vi "MultiTool-Track-Generate-ndipolarisFileOutput-Q-vectors-Accepts Joystick mod10Feb2018.vi"() -> ()   [LabVIEW 2013]
panel:
  out "TIME":string
  out "bytes written":i32
  out "Return time string":string
  out "Length":u8
  out "Command":u8
  out "Tool 2":T1={"Port Handle"="", "Frame Number"=0, "Tx"=0.0, "Ty"=0.0, "Tz"=0.0, "Q0"=0.0, "Qx"=0.0, "Qy"=0.0, "Qz"=0.0, "Deviation"=0.0, " Markers Missing"=TRUE, "Out of Volume"=TRUE} {"Deviation" format="%#.4f"; "Qz" format="%#.4f"; "Qy" format="%#.4f"; "Qx" format="%#.4f"; "Q0" format="%#.4f"; "Tz" format="%#.2f"; "Ty" format="%#.2f"; "Tx" format="%#.2f"}
  in  "Location of ROM File for Tool 2":path=path "C:/Program Files (x86)/Northern Digital Inc/8700339.rom"
  in  "NDI  Running":bool=TRUE
  out "Stop Reading":bool=TRUE
  out "Start Reading":bool
  out "Object Identifier":string="0"
  in  "Track Outside Measurement Volume? (F:No)":bool
  in  "Track Stray Markers? (F:No)":bool
  out "Tool 1":T1={"Port Handle"="", "Frame Number"=0, "Tx"=0.0, "Ty"=0.0, "Tz"=0.0, "Q0"=0.0, "Qx"=0.0, "Qy"=0.0, "Qz"=0.0, "Deviation"=0.0, " Markers Missing"=TRUE, "Out of Volume"=TRUE} {"Deviation" format="%#.4f"; "Qz" format="%#.4f"; "Qy" format="%#.4f"; "Qx" format="%#.4f"; "Q0" format="%#.4f"; "Tz" format="%#.2f"; "Ty" format="%#.2f"; "Tx" format="%#.2f"}
  out "TCP loop":i32
  in  "TCP Server Running":bool=TRUE
  in  "Output Directory":path=path "C:/Users/Diogo/Desktop/NDI-Labview Gripper"
  out "NDI Loop":i32
  in  "VISA resource name":refnum<visa-resource-name>="COM8"
  in  "Reset? (T:Yes)":bool=TRUE
  in  "Location of ROM File for Tool 1":path=path "C:/Program Files (x86)/Northern Digital Inc/8700449.rom"
  in  "Serial Configuration":T2={"Baud Rate (9600)"=9600, "Flow Control (0:None)"=0, "Parity"=0, "Data Bits"=8, "Stop Bits"=10} {"Stop Bits" items=["1.0"=10, "2.0"=20]; "Parity" items=["None", "Odd", "Even"]; "Flow Control (0:None)" items=["None", "XON/XOFF"]; "Baud Rate (9600)" items=["9600"=9600, "14.4k"=14400, "19.2k"=19200, "38.4k"=38400, "57.6k "=57600, "115.2k"=115200]}
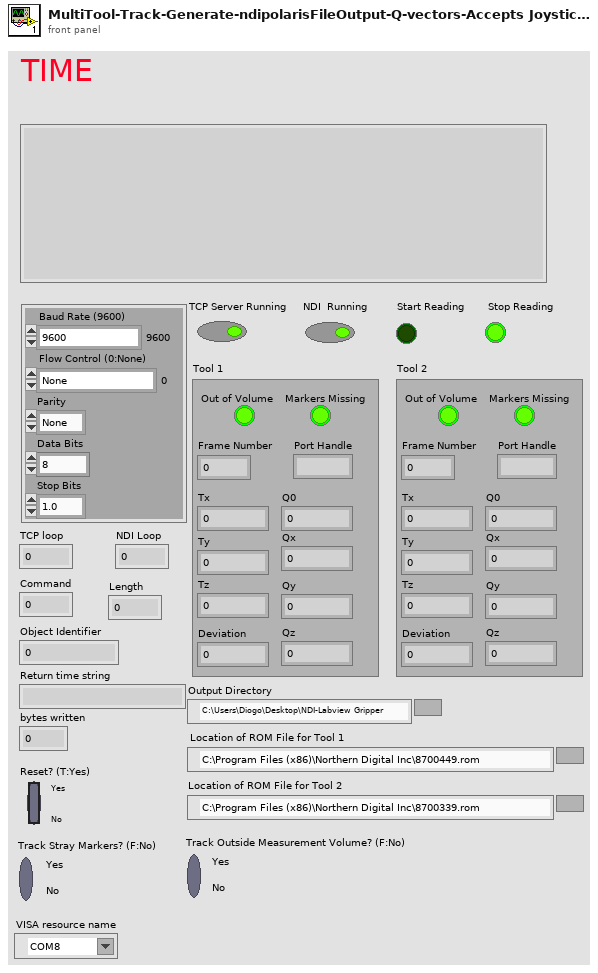
[diagram p1: front panel]
types:
  T1 = cluster{"Port Handle":string, "Frame Number":i32, "Tx":dbl, "Ty":dbl, "Tz":dbl, "Q0":dbl, "Qx":dbl, "Qy":dbl, "Qz":dbl, "Deviation":dbl, " Markers Missing":bool, "Out of Volume":bool}
  T2 = cluster{"Baud Rate (9600)":u32, "Flow Control (0:None)":u16, "Parity":u16, "Data Bits":u16, "Stop Bits":u16}
  T3 = cluster{"Port Handle":string, "Frame Number":u32, "Tx":dbl, "Ty":dbl, "Tz":dbl, "Q0":dbl, "Qx":dbl, "Qy":dbl, "Qz":dbl, "Deviation":dbl, "Missing?":bool, "Out of Volume?":bool}[]
  T4 = cluster{"Transformations[0]":cluster{"Port Handle":string, "Frame Number":u32, "Tx":dbl, "Ty":dbl, "Tz":dbl, "Q0":dbl, "Qx":dbl, "Qy":dbl, "Qz":dbl, "Deviation":dbl, "Missing?":bool, "Out of Volume?":bool}, "Transformations[1]":cluster{"Port Handle":string, "Frame Number":u32, "Tx":dbl, "Ty":dbl, "Tz":dbl, "Q0":dbl, "Qx":dbl, "Qy":dbl, "Qz":dbl, "Deviation":dbl, "Missing?":bool, "Out of Volume?":bool}, "Transformations[2]":cluster{"Port Handle":string, "Frame Number":u32, "Tx":dbl, "Ty":dbl, "Tz":dbl, "Q0":dbl, "Qx":dbl, "Qy":dbl, "Qz":dbl, "Deviation":dbl, "Missing?":bool, "Out of Volume?":bool}, "Transformations[3]":cluster{"Port Handle":string, "Frame Number":u32, "Tx":dbl, "Ty":dbl, "Tz":dbl, "Q0":dbl, "Qx":dbl, "Qy":dbl, "Qz":dbl, "Deviation":dbl, "Missing?":bool, "Out of Volume?":bool}, "Transformations[4]":cluster{"Port Handle":string, "Frame Number":u32, "Tx":dbl, "Ty":dbl, "Tz":dbl, "Q0":dbl, "Qx":dbl, "Qy":dbl, "Qz":dbl, "Deviation":dbl, "Missing?":bool, "Out of Volume?":bool}, "Transformations[5]":cluster{"Port Handle":string, "Frame Number":u32, "Tx":dbl, "Ty":dbl, "Tz":dbl, "Q0":dbl, "Qx":dbl, "Qy":dbl, "Qz":dbl, "Deviation":dbl, "Missing?":bool, "Out of Volume?":bool}, "Transformations[6]":cluster{"Port Handle":string, "Frame Number":u32, "Tx":dbl, "Ty":dbl, "Tz":dbl, "Q0":dbl, "Qx":dbl, "Qy":dbl, "Qz":dbl, "Deviation":dbl, "Missing?":bool, "Out of Volume?":bool}, "Transformations[7]":cluster{"Port Handle":string, "Frame Number":u32, "Tx":dbl, "Ty":dbl, "Tz":dbl, "Q0":dbl, "Qx":dbl, "Qy":dbl, "Qz":dbl, "Deviation":dbl, "Missing?":bool, "Out of Volume?":bool}, "Transformations[8]":cluster{"Port Handle":string, "Frame Number":u32, "Tx":dbl, "Ty":dbl, "Tz":dbl, "Q0":dbl, "Qx":dbl, "Qy":dbl, "Qz":dbl, "Deviation":dbl, "Missing?":bool, "Out of Volume?":bool}}
  T5 = cluster{"Port Handle":string, "Frame Number":u32, "Tx":dbl, "Ty":dbl, "Tz":dbl, "Q0":dbl, "Qx":dbl, "Qy":dbl, "Qz":dbl, "Deviation":dbl, "Missing?":bool, "Out of Volume?":bool}
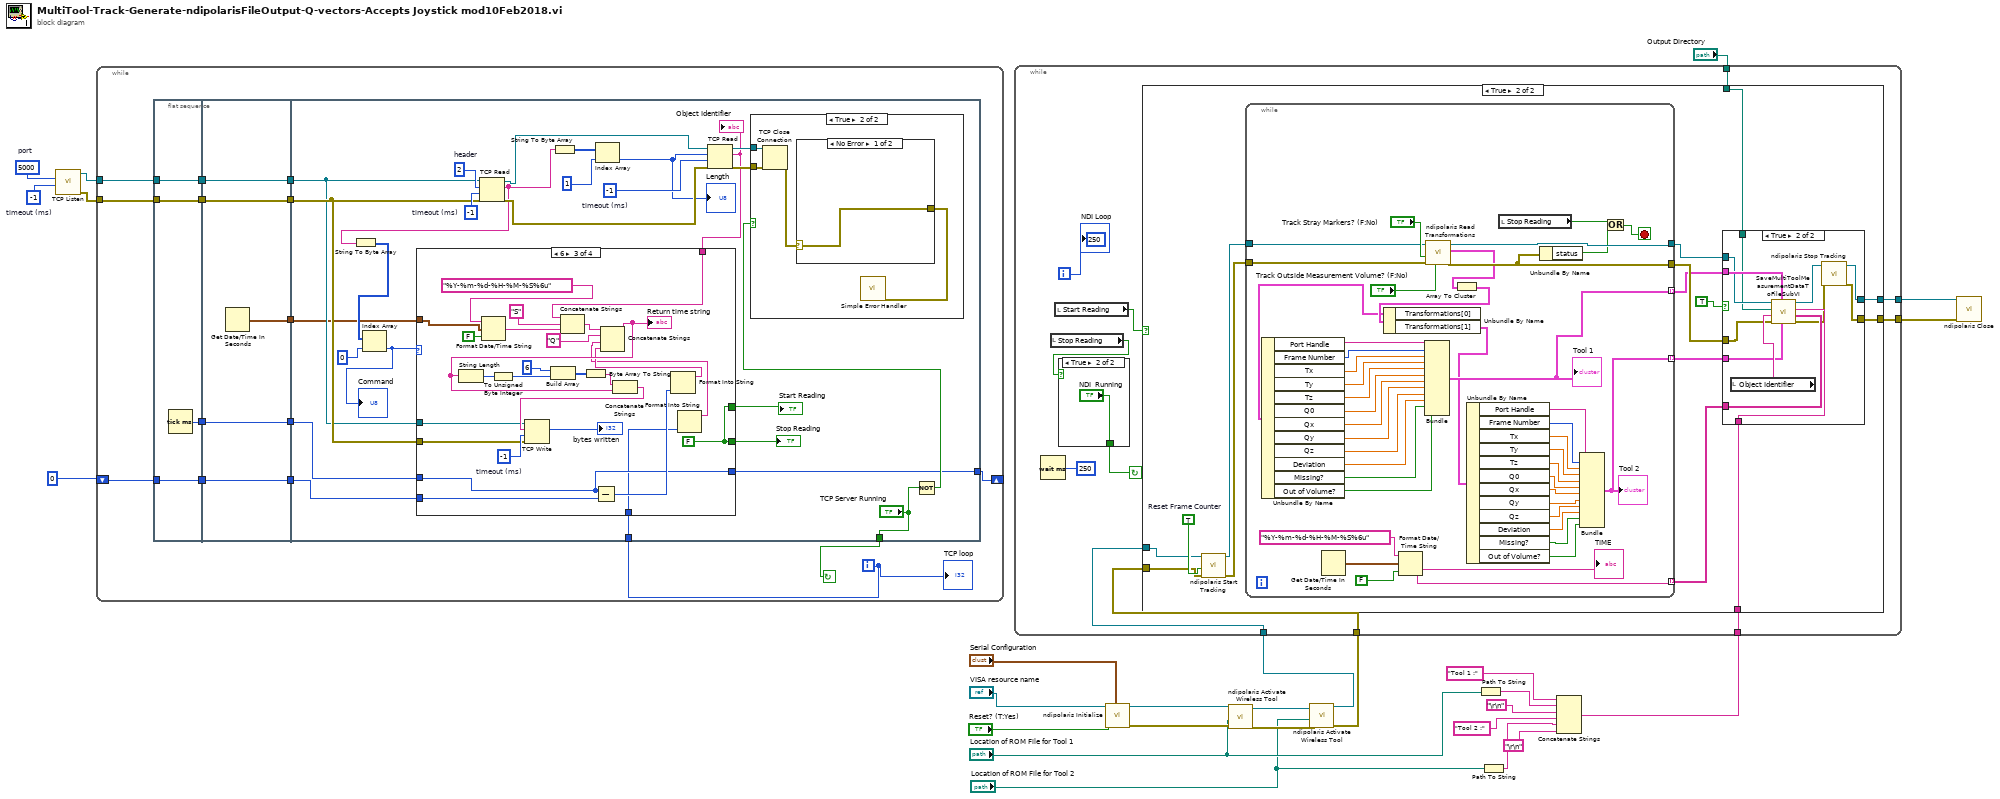
[diagram p0: block diagram]
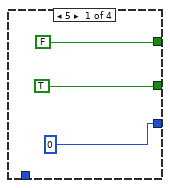
[diagram p2: hidden frame]
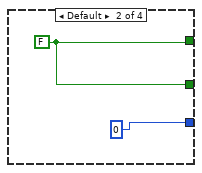
[diagram p3: hidden frame]
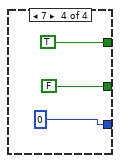
[diagram p4: hidden frame]
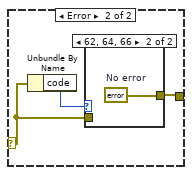
[diagram p6: hidden frame]
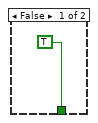
[diagram p8: hidden frame]
diagram:
  w26 = u16 5000  # port
  w25 = i8 -1  # timeout (ms)
  n1 = call <vilib>:"TCP Listen.vi"("timeout ms (wait forever: -1)"=w25, "port"=w26) -> ("error out"=w20:errorcluster, "connection ID"=w21:refnum<k5>)  [unwired: 5 in, 3 out]
  n2 = while {
    tunnel: w21 -> [w39]
    tunnel: w20 -> [w40]
    shift-right: [w33] -> _
    shift-left: u32 0 -> [w35]
    i -> [w27]
    stop <- w41 continue-if-true
    n3 = flat-sequence {
      tunnel: w35 -> [w43]
      tunnel: w39 -> [w44]
      tunnel: w40 -> [w45]
      tunnel: [w45] -> w32
      tunnel: [w44] -> w31
      tunnel: [w43] -> w30
      tunnel: [w42] -> w28
      tunnel: [w50] -> w38
      tunnel: [w49] -> w37
      tunnel: [w48] -> w36
      tunnel: [w47] -> w34
      tunnel: w32 -> [w50]
      tunnel: w31 -> [w49]
      tunnel: w30 -> [w47]
      tunnel: [w46] -> w29
      tunnel: w28 -> [w46]
      tunnel: ["TCP Server Running"] -> w41
      tunnel: w38 -> [w58]
      tunnel: w37 -> [w56]
      tunnel: w36 -> [w55]
      tunnel: w34 -> [w54]
      tunnel: [w53] -> w33
      tunnel: w29 -> [w52]
      tunnel: w27 -> [w51]
      frame #0 {
        n4 = Tick Count (ms)() -> (millisecond timer value=w42:u32)
      }
      frame #1 {
        n5 = Get Date/Time In Seconds() -> (seconds since 1Jan1904=w48:timestamp)
      }
      frame #2 {
        w72 = i8 -1  # timeout (ms)
        w75 = i8 -1  # timeout (ms)
        w76 = i8 2  # header
        n6 = TCP Read(connection ID=w56, bytes to read=w76, error in (no error)=w58, 9:w75) -> (connection ID out=w74:refnum<k5>, data out=w63:string, error out=w73:errorcluster)  [unwired: 1 in]
        n7 = String To Byte Array(string=w63) -> (unsigned byte array=w66:u8[])
        n8 = Index Array(array=w66, index=0) -> (element=w59:u8)
        "Command" <- w59
        n9 = String To Byte Array(string=w63) -> (unsigned byte array=w65:u8[])
        n10 = Index Array(array=w65, index=1) -> (element=w62:u8)
        "Length" <- w62
        n11 = TCP Read(connection ID=w74, bytes to read=w62, error in (no error)=w73, 9:w72) -> (connection ID out=w71:refnum<k5>, data out=w57:string, error out=w70:errorcluster)  [unwired: 1 in]
        "Object Identifier" <- w57
        n12 = case shown="6" w59 {
          tunnel: [FALSE w81 w93 TRUE] -> w69
          tunnel: [TRUE w81 w93 FALSE] -> w68
          tunnel: w58 -> [_ _ w96 _]
          tunnel: w57 -> [_ _ w95 _]
          tunnel: w56 -> [_ _ w94 _]
          tunnel: w55 -> [_ _ w92 _]
          tunnel: w54 -> [_ _ w86 _]
          tunnel: [u32 0 u32 0 w85 u32 0] -> w53
          tunnel: w52 -> [_ _ w85 _]
          tunnel: w51 -> [_ _ w82 _]
          frame 5 {
          }
          frame Default {
            w81 = FALSE
          }
          frame 6 {
            w104 = i8 -1  # timeout (ms)
            w93 = FALSE
            n13 = Format Date/Time String(time format string (%c)="%Y-%m-%d-%H-%M-%S%6u", seconds (now)=w92, UTC format=FALSE) -> (date/time string=w107:string)
            n14 = Concatenate Strings(w95, "S", w107) -> (w91:string)
            n15 = Subtract(x=w85, y=w86) -> (x-y=w87:u32)
            n16 = Format Into String(w87) -> (resulting string=w84:string)  [unwired: 3 in, 1 out]
            n17 = Format Into String(w82) -> (resulting string=w83:string)  [unwired: 3 in, 1 out]
            n18 = Concatenate Strings(w91, "Q", w83, w84) -> (w89:string)
            "Return time string" <- w89
            n19 = String Length(string=w89) -> (length=w101:i32)
            n20 = To Unsigned Byte Integer(number=w101) -> (unsigned 8bit integer=w100:u8)
            n21 = Build Array(u8 6, w100) -> (w98:u8[])
            n22 = Byte Array To String(unsigned byte array=w98) -> (string=w103:string)
            n23 = Concatenate Strings(w103, w89) -> (w97:string)
            n24 = TCP Write(connection ID=w94, data in=w97, error in (no error)=w96, 9:w104) -> (bytes written=→"bytes written":i32)  [unwired: 2 out]
          }
          frame 7 {
          }
        }
        "Start Reading" <- w69
        "Stop Reading" <- w68
        n25 = Not(x="TCP Server Running") -> (.not. x?=w60:bool)
        n26 = case shown="True" w60 {
          tunnel: w71 -> [_ w112]
          tunnel: w70 -> [_ w111]
          frame False {
          }
          frame True {
            n27 = TCP Close Connection(connection ID=w112, error in (no error)=w111) -> (error out=w113:errorcluster)  [unwired: 1 in, 1 out]
            n28 = case shown="No Error" w113 {
              selector: w113 -> [w115 w117]
              tunnel: [w115 w116] -> w114
              frame No Error {
              }
              frame Error {
                n29 = Unbundle By Name(w117) -> ("code"=w118:i32)
                n30 = case shown="62, 64, 66" w118 {
                  tunnel: w117 -> [w119 _]
                  tunnel: [w119 w120] -> w116
                  frame Default {
                  }
                  frame 62, 64, 66 {
                    w120 = errorcluster {"status"=FALSE, "code"=0, "source"=""}  # No error
                  }
                }
              }
            }
            n31 = call <vilib>:"Simple Error Handler.vi"("error in (no error)"=w114) -> ()  [unwired: 1 in, 8 out]
          }
        }
      }
    }
    "TCP loop" <- w27
  }
  n32 = call <instrlib>:"ndipolaris Initialize.vi"("Serial Configuration"="Serial Configuration", "Reset? (T: Yes)"="Reset? (T:Yes)", "VISA resource name"="VISA resource name") -> ("error out"=w16:errorcluster, "VISA resource name out"=w17:refnum<visa-resource-name>)  [unwired: 7 in]
  n33 = call <instrlib>:"ndipolaris Activate Wireless Tool.vi"("error in (no error)"=w16, "Location of ROM File for Tool"="Location of ROM File for Tool 1", "VISA resource name"=w17) -> ("error out"=w14:errorcluster, "VISA resource out"=w15:refnum<visa-resource-name>)  [unwired: 6 in, 1 out]
  n34 = call <instrlib>:"ndipolaris Activate Wireless Tool.vi"("error in (no error)"=w14, "Location of ROM File for Tool"="Location of ROM File for Tool 2", "VISA resource name"=w15) -> ("error out"=w3:errorcluster, "VISA resource out"=w4:refnum<visa-resource-name>)  [unwired: 6 in, 1 out]
  n35 = Path To String(path="Location of ROM File for Tool 1") -> (string=w10:string)
  n36 = Path To String(path="Location of ROM File for Tool 2") -> (string=w8:string)
  n37 = Concatenate Strings("Tool 1 :" ("string"), w10, "\r\n", "Tool 2 :" ("string"), w8, "\r\n") -> (w18:string)
  n38 = while {
    tunnel: [w130] -> w2
    tunnel: "Output Directory" -> [w129]
    tunnel: [w128] -> w1
    tunnel: w18 -> [w124]
    tunnel: w4 -> [w122]
    tunnel: w3 -> [w121]
    i -> [w131]
    stop <- w123 continue-if-true
    (unwired) u8 250
    n39 = Wait (ms)(milliseconds to wait=u32 250) -> ()  [unwired: 1 out]
    n40 = local read "Stop Reading"() -> (w125:bool)
    n41 = local read "Start Reading"() -> (w126:bool)
    n42 = case shown="True" w125 {
      tunnel: [TRUE "NDI  Running"] -> w123
      frame False {
      }
      frame True {
      }
    }
    n43 = case shown="True" w126 {
      tunnel: w122 -> [w135 w137]
      tunnel: [w135 w148] -> w130
      tunnel: w129 -> [_ w150]
      tunnel: [w134 w147] -> w128
      tunnel: w124 -> [_ w142]
      tunnel: w121 -> [w134 w136]
      frame False {
      }
      frame True {
        w138 = TRUE  # Reset Frame Counter
        n44 = call <instrlib>:"ndipolaris Start Tracking.vi"("error in (no error)"=w136, "Reset Frame Counter? (F:No)"=w138, "VISA resource name"=w137) -> ("error out"=w140:errorcluster, "VISA resource out"=w139:refnum<visa-resource-name>)  [unwired: 7 in]
        n45 = while {
          tunnel: [w206] -> w144
          tunnel: [w205] -> w149
          tunnel: [w182] -> w145 mode=indexing
          tunnel: [w183] -> w146 mode=indexing
          tunnel: w139 -> [w181]
          tunnel: w140 -> [w180]
          tunnel: [w165] -> w141 mode=indexing
          stop <- w207 stop-if-true
          n46 = Get Date/Time In Seconds() -> (seconds since 1Jan1904=w186:timestamp)
          n47 = Format Date/Time String(time format string (%c)="%Y-%m-%d-%H-%M-%S%6u", seconds (now)=w186, UTC format=FALSE) -> (date/time string=w183:string)
          "TIME" <- w183
          n48 = call <instrlib>:"ndipolaris Read Transformations.vi"("Track Outside Measurement Volume? (F:No)"="Track Outside Measurement Volume? (F:No)", "error in (no error)"=w180, "Track Stray Markers? (F:No)"="Track Stray Markers? (F:No)", "VISA resource name"=w181) -> ("error out"=w205:errorcluster, "Transformations"=w190:T3, "VISA resource out"=w206:refnum<visa-resource-name>)  [unwired: 4 in, 1 out]
          n49 = Array To Cluster(array=w190) -> (cluster=w201:T4)
          n50 = Unbundle By Name(w201) -> ("Transformations[0]"=w200:T5, "Transformations[1]"=w178:T5)
          n51 = Unbundle By Name(w200) -> ("Port Handle"=w199:string, "Frame Number"=w198:u32, "Tx"=w197:dbl, "Ty"=w196:dbl, "Tz"=w195:dbl, "Q0"=w194:dbl, "Qx"=w193:dbl, "Qy"=w192:dbl, "Qz"=w191:dbl, "Deviation"=w189:dbl, "Missing?"=w188:bool, "Out of Volume?"=w187:bool)
          n52 = Bundle("Port Handle"=w199, "Frame Number"=w198, "Tx"=w197, "Ty"=w196, "Tz"=w195, "Q0"=w194, "Qx"=w193, "Qy"=w192, "Qz"=w191, "Deviation"=w189, "Missing?"=w188, "Out of Volume?"=w187) -> (w182:T5)  [unwired: 1 in]
          "Tool 1" <- w182
          n53 = Unbundle By Name(w178) -> ("Port Handle"=w177:string, "Frame Number"=w176:u32, "Tx"=w175:dbl, "Ty"=w174:dbl, "Tz"=w173:dbl, "Q0"=w172:dbl, "Qx"=w171:dbl, "Qy"=w170:dbl, "Qz"=w169:dbl, "Deviation"=w168:dbl, "Missing?"=w167:bool, "Out of Volume?"=w166:bool)
          n54 = local read "Stop Reading"() -> (w179:bool)
          n55 = Unbundle By Name(w205) -> ("status"=w204:bool)
          n56 = Bundle("Port Handle"=w177, "Frame Number"=w176, "Tx"=w175, "Ty"=w174, "Tz"=w173, "Q0"=w172, "Qx"=w171, "Qy"=w170, "Qz"=w169, "Deviation"=w168, "Missing?"=w167, "Out of Volume?"=w166) -> (w165:T5)  [unwired: 1 in]
          "Tool 2" <- w165
          n57 = Or(x=w179, y=w204) -> (x .or. y?=w207:bool)
        }
        n58 = case shown="True" TRUE {
          tunnel: w150 -> [_ w162]
          tunnel: w149 -> [w151 w160]
          tunnel: [w152 w153] -> w148
          tunnel: [w151 w154] -> w147
          tunnel: w146 -> [_ w159]
          tunnel: w145 -> [_ w164]
          tunnel: w144 -> [w152 w163]
          tunnel: w142 -> [_ w158]
          tunnel: w141 -> [_ w157]
          frame False {
          }
          frame True {
            n59 = local read "Object Identifier"() -> (w161:string)
            n60 = call "SaveMultiToolMeasurementDataToFileSubVI.vi"("Array of Time for Measurement"=w159, "NDI Tool"=w158, "Array - Transformations of Tool 2"=w157, "Array - Transformations of Tool 1"=w164, "error in (no error)"=w160, "Object number"=w161, "Output Directory"=w162, "VISA Refnum in"=w163) -> ("error out"=w155:errorcluster, "VISA Refnum out"=w156:refnum<visa-resource-name>)
            n61 = call <instrlib>:"ndipolaris Stop Tracking.vi"("error in (no error)"=w155, "VISA resource name"=w156) -> ("error out"=w154:errorcluster, "VISA resource out"=w153:refnum<visa-resource-name>)  [unwired: 8 in]
          }
        }
      }
    }
    "NDI Loop" <- w131
  }
  n62 = call <instrlib>:"ndipolaris Close.vi"("error in (no error)"=w1, "VISA resource name"=w2) -> ()  [unwired: 9 in, 1 out]
